vi "Copy 7zSD.SFX.vi"(8 "error in (no error)":errorcluster, 11 "PostBuildSupport in":refnum<class "PostBuildSupport.lvclass">) -> (0 "error out":errorcluster, 3 "PostBuildSupport out":refnum<class "PostBuildSupport.lvclass">)   [LabVIEW 2016, in "PostBuildSupport.lvclass"]
uses:
  PostBuildSupport.lvclass
  PostBuildSupport.lvclass/PostBuildSupport.ctl
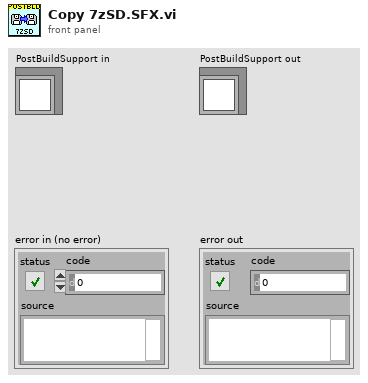
[diagram p1: front panel]
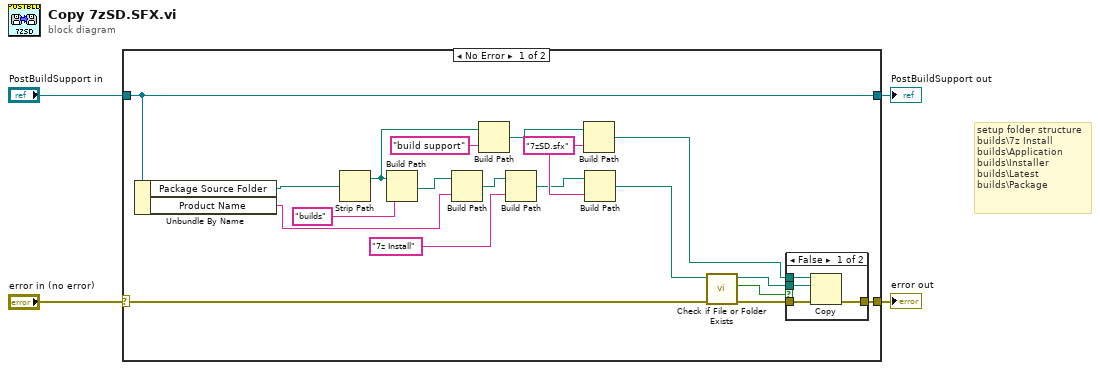
[diagram p0: block diagram]
diagram:
  # "setup folder structure\nbuilds\\7z Install\nbuilds\\Application\nbuilds\\Installer\nbuilds\\Latest\nbuilds\\Package"
  n1 = case shown="No Error" "error in (no error)" {
    selector: "error in (no error)" -> [w6 w29]
    tunnel: [w19 w29] -> w4
    tunnel: "PostBuildSupport in" -> [w5 w30]
    tunnel: [w5 w30] -> w1
    frame No Error {
      w13 = "7zSD.sfx" ("name or relative path")
      n2 = Unbundle By Name(w5) -> ("Package Source Folder"=w21:path, "Product Name"=w20:string)
      n3 = Strip Path(path=w21) -> (stripped path=w14:path)  [unwired: 1 out]
      n4 = Build Path(base path=w14, name or relative path="builds") -> (appended path=w22:path)
      n5 = Build Path(base path=w22, name or relative path=w20) -> (appended path=w16:path)
      n6 = Build Path(base path=w14, name or relative path="build support") -> (appended path=w17:path)
      n7 = Build Path(base path=w16, name or relative path="7z Install") -> (appended path=w12:path)
      n8 = Build Path(base path=w17, name or relative path=w13) -> (appended path=w7:path)
      n9 = Build Path(base path=w12, name or relative path=w13) -> (appended path=w11:path)
      n10 = call <vilib>:"Check if File or Folder Exists.vi"("error in (no error)"=w6, "path"=w11) -> ("error out"=w9:errorcluster, "file or folder exists?"=w8:bool, "dup path"=w10:path)  [unwired: 7 in]
      n11 = case shown="False" w8 {
        tunnel: [w27 w28] -> w19
        tunnel: w7 -> [w26 _]
        tunnel: w10 -> [w25 _]
        tunnel: w9 -> [w24 w28]
        frame False {
          n12 = Copy(8:w24, 10:w25, 11:w26) -> (0:w27:errorcluster)  [unwired: 2 in, 2 out]
        }
        frame True {
        }
      }
    }
    frame Error {
    }
  }
  "error out" <- w4
  "PostBuildSupport out" <- w1
